vi "principal.vi"() -> ()   [LabVIEW 2020]
uses:
  <vilib>/vision/Pattern Matching.llb/IMAQ GM Match Report.ctl
panel:
  in  "?":bool
  out "Aprovado":bool
  out "Image Out":T1(plugin-control)
  out "Number of Matches":i32
  out "Matches (Pattern Matching 1)":T2[](array[typedef]) {"Correlation Score" format="%.2f"; "Target Template Curve Score" format="%.2f"; "Template Target Curve Score" format="%.2f"; "Bounding Box"."y" format="%.2f"; "Bounding Box"."x" format="%.2f"; "Position"."y" format="%.2f"; "Position"."x" format="%.2f"; "Score" format="%.2f"; "Scale" format="%.2f"; "Angle" format="%.2f"; "Occlusion %" format="%.2f"}
  out "error out":errorcluster
  in  "error in":errorcluster
  # "Teste de Pino"
  # "Sample\nNegativa"
  # "Sample \nPositiva"
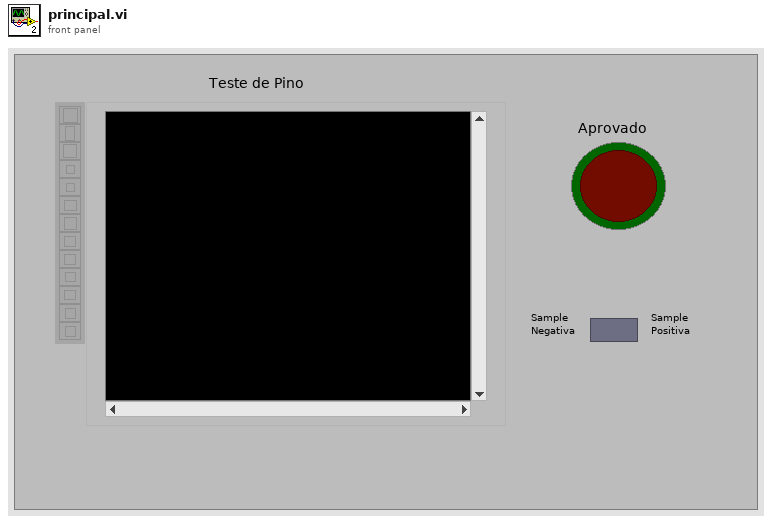
[diagram p1: front panel]
types:
  T1 = typedef "IMAQ Image.ctl" = refnum<image>
  T2 = typedef "IMAQ GM Match Report.ctl" = cluster{"Position":cluster{"x":sgl, "y":sgl}, "Angle":sgl, "Scale":sgl, "Score":sgl, "Bounding Box":cluster{"x":sgl, "y":sgl}[], "Contrast Reversed":bool, "Occlusion %":sgl, "Template Target Curve Score":sgl, "Target Template Curve Score":sgl, "Correlation Score":sgl}
  T3 = cluster{"Global Rectangle":i32[], "Contours":cluster{"ID":enum32{"External", "Internal"}, "Type":u32, "Coordinates":i32[]}[]}
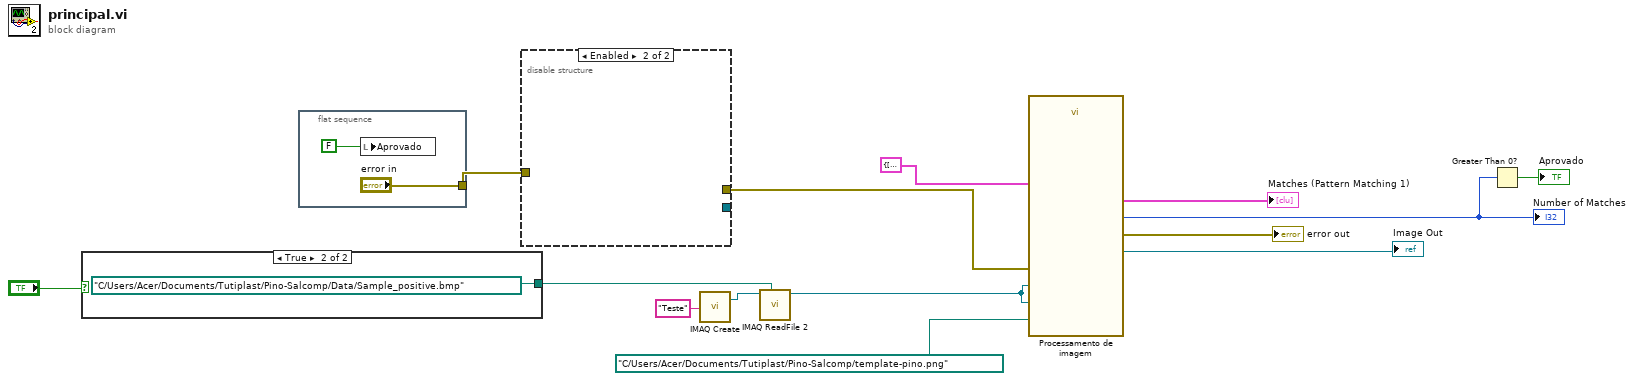
[diagram p0: block diagram]
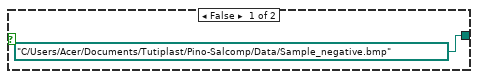
[diagram p2: hidden frame]
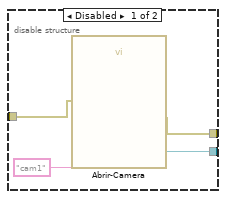
[diagram p3: hidden frame]
diagram:
  n1 = case shown="True" "?" {
    tunnel: [path "C:/Users/Acer/Documents/Tutiplast/Pino-Salcomp/Data/Sample_negative.bmp" ("File Path") path "C:/Users/Acer/Documents/Tutiplast/Pino-Salcomp/Data/Sample_positive.bmp" ("File Path")] -> w3
    frame False {
    }
    frame True {
    }
  }
  n2 = flat-sequence {
    tunnel: ["error in"] -> w13
    frame #0 {
      n3 = local write "Aprovado"(FALSE) -> ()
    }
  }
  n4 = disable-structure shown="Enabled" {
    disable-tunnel: w13 -> [w22 _]
    disable-tunnel: [w20 _] -> w12
    disable-tunnel: [w19 _] -> _
    frame Disabled {
      n5 = call "Abrir-Camera.vi"("Interface Name"="cam1", "error in"=w22) -> ("Image Out"=w19:T1, "error out"=w20:errorcluster)  [unwired: 24 in]
    }
    frame Enabled {
    }
  }
  n6 = call "IMAQ Create"("Image Name"="Teste") -> ("New Image"=w4:T1)  [unwired: 4 in, 1 out]
  n7 = call "IMAQ ReadFile 2"("File Path"=w3, "Image"=w4) -> ("Image Out"=w2:T1)  [unwired: 5 in, 4 out]
  n8 = call "Processamento de imagem.vi"("Image In"=w2, "Image Dst"=w2, "ROI Descriptor (Pattern Matching 1)"=T3 {"Global Rectangle"=[20, 20, 2284, 1516], "Contours"=[{"ID"=enum."External", "Type"=3, "Coordinates"=[20, 20, 2284, 1516]}]}, "Template File Path"=path "C:/Users/Acer/Documents/Tutiplast/Pino-Salcomp/template-pino.png", "error in"=w12) -> ("Image Out"=→"Image Out":T1, "Matches (Pattern Matching 1)"=→"Matches (Pattern Matching 1)":T2[], "Number of Matches (Pattern Matching 1)"=w7:i32, "error out"=→"error out":errorcluster)  [unwired: 19 in]
  "Number of Matches" <- w7
  n9 = Greater Than 0?(x=w7) -> (x > 0?=→"Aprovado":bool)
